vi "ErrorHandler.vi"(8 "error in (no error)":errorcluster, 11 "ModuleAdmin":refnum<class "ModuleAdmin.lvclass">) -> (0 "error out":errorcluster, 3 "ModuleAdmin Out":refnum<class "ModuleAdmin.lvclass">)   [LabVIEW 2018, in "SpecAnPlugins.lvlib"]
doc: "Handle an error by enqueueing an \"Error\" message to the front of the queue."
uses:
  SpecAnPlugins/SpecAnPlugins.lvlib
  <userlib>/NIST/ModuleAdminLib/ModuleAdmin/ModuleAdmin.lvclass
panel:
  in  "Message (Error)":string="Error"
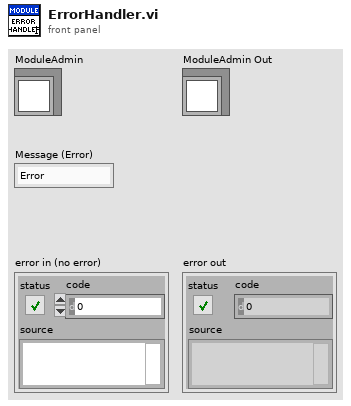
[diagram p1: front panel]
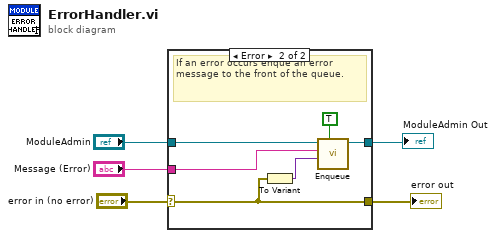
[diagram p0: block diagram]
diagram:
  n1 = case shown="Error" "error in (no error)" {
    selector: "error in (no error)" -> [w6 w8]
    tunnel: "Message (Error)" -> [_ w12]
    tunnel: [w7 w10] -> w3
    tunnel: "ModuleAdmin" -> [w7 w9]
    tunnel: [w6 w8] -> w1
    frame No Error {
    }
    frame Error {
      # "If an error occurs enque an error message to the front of the queue."
      n2 = To Variant(anything=w8) -> (Variant=w13:variant)
      n3 = call "Enqueue.vi"("Priority (F)"=TRUE, "Message Data"=w13, "Message"=w12, "ModuleAdmin"=w9) -> ("ModuleAdmin Out"=w10:refnum<class "ModuleAdmin.lvclass">)  [unwired: 6 in, 1 out]
    }
  }
  "error out" <- w1
  "ModuleAdmin Out" <- w3
